vi "Image Paths.vi"(11 "base path":path) -> (2 "Line Image Path":path, 3 "Original Image Path":path)   [LabVIEW 2011]
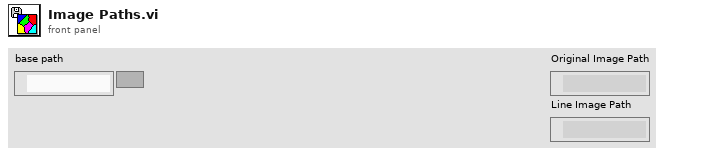
[diagram p1: front panel]
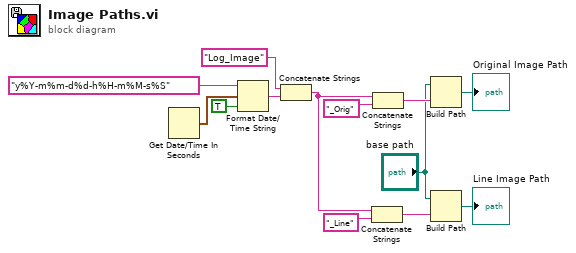
[diagram p0: block diagram]
diagram:
  n1 = Get Date/Time In Seconds() -> (seconds since 1Jan1904=w10:timestamp)
  n2 = Format Date/Time String(time format string (%c)="y%Y-m%m-d%d-h%H-m%M-s%S", seconds (now)=w10, UTC format=TRUE) -> (date/time string=w12:string)
  n3 = Concatenate Strings("Log_Image", w12) -> (w8:string)
  n4 = Concatenate Strings(w8, "_Line") -> (w7:string)
  n5 = Concatenate Strings(w8, "_Orig") -> (w6:string)
  n6 = Build Path(base path="base path", name or relative path=w6) -> (appended path=→"Original Image Path":path)
  n7 = Build Path(base path="base path", name or relative path=w7) -> (appended path=→"Line Image Path":path)
